vi "Bundle Script_Cluster Terminal Bundle.vi"(4 "Hide Full Names":bool=TRUE, 6 "Object Placement":enum32{"Choice 1", "Choice 2"}(radio), 8 "error in":errorcluster, 10 "Selected Items Tags":string[](array[string]), 11 "Affected Items":T1) -> (0 "error out":errorcluster, 2 "Objects":refnum<vi>[](array[refnum]))   [LabVIEW 2023]
uses:
  top/BundleMagic.ctl
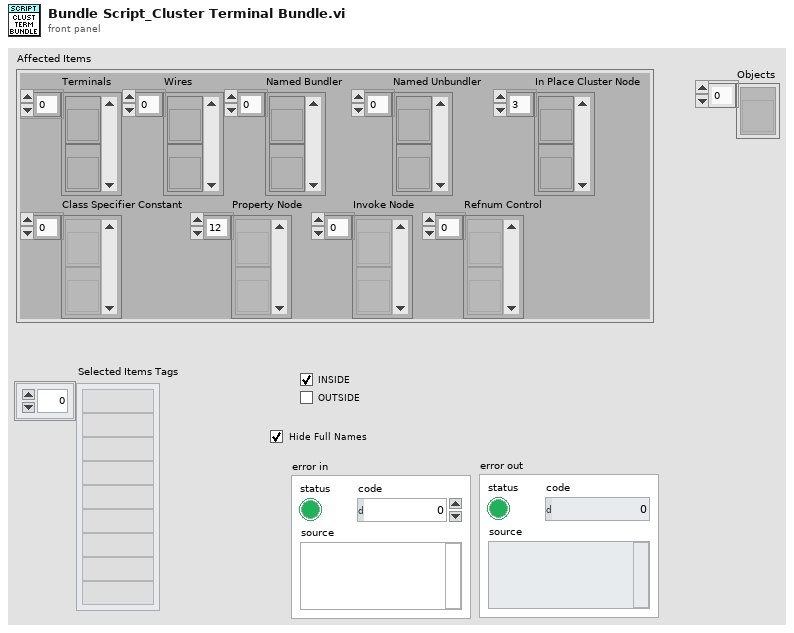
[diagram p1: front panel]
types:
  T1 = typedef "BundleMagic.ctl" = cluster{"Terminals":refnum<vi>[], "Wires":refnum<vi>[], "Named Bundler":refnum<vi>[], "Named Unbundler":refnum<vi>[], "In Place Cluster Node":refnum<vi>[], "Class Specifier Constant":refnum<vi>[], "Property Node":refnum<vi>[], "Invoke Node":refnum<vi>[], "Refnum Control":refnum<vi>[]}
  T2 = enum32{"Top Edges", "Vertical Centers", "Bottom Edges", "Left Edges", "Horizontal Centers", "Right Edges"}
  T3 = cluster{"Tunnel Ref":refnum<vi>, "On Tunnel?":bool, "Placement":enum32{"Choice 1", "Choice 2"}, "Tunnel Is Indexing?":bool, "Diagram":refnum<vi>, "Position":cluster{"Refnum":refnum<vi>, "Relative Direction":enum32{"Right", "Left", "Top", "Bottom", "Top Right", "Top Left", "Bottom Right", "Bottom Left"}, "Point32":cluster{"Horizontal":i32, "Vertical":i32}}, "Chosen Terminal":refnum<vi>, "Is Refnum?":bool, "Is Cluster?":bool, "Is Source?":bool, "Tunnel Direction":enum16{"In-Going", "Out-Going"}, "Tunnel Position":enum16{"Left", "Top", "Right", "Bottom"}, "Is Inner?":bool, "Terminal Is Indexing?":bool}
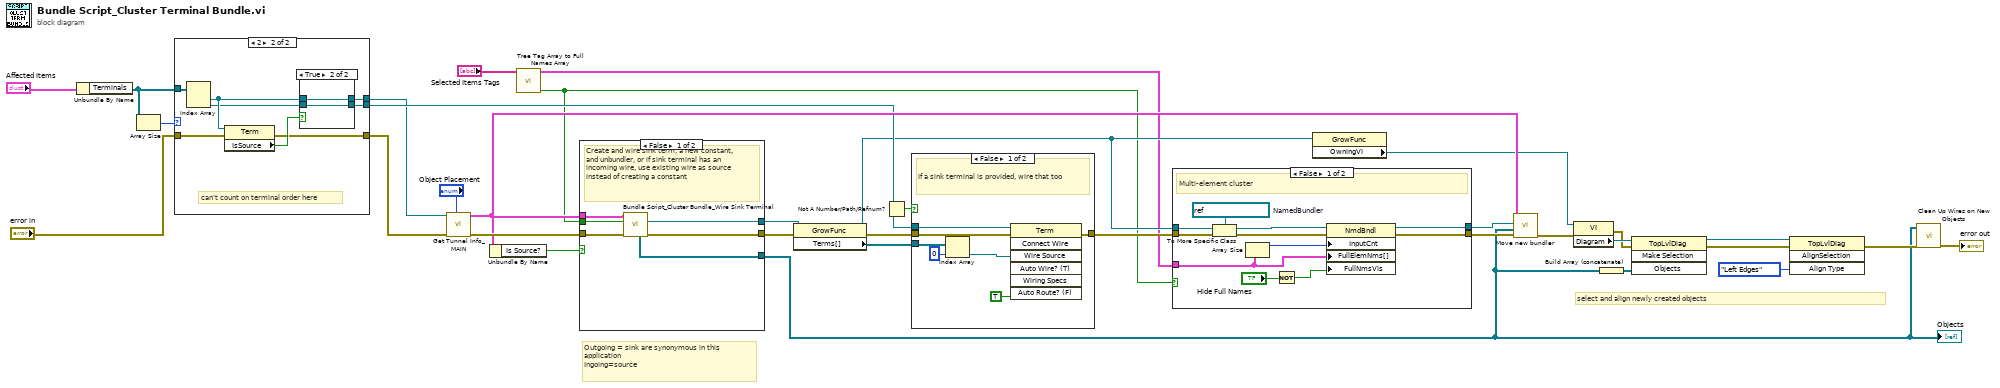
[diagram p0: block diagram]
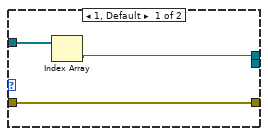
[diagram p2: hidden frame]
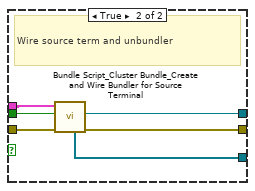
[diagram p4: hidden frame]
diagram:
  # "Outgoing = sink are synonymous in this application\nIngoing=source"
  # "select and align newly created objects"
  n1 = Unbundle By Name("Affected Items") -> ("Terminals"=w14:refnum<vi>[])
  n2 = Array Size(array=w14) -> (size(s)=w13:i32)
  n3 = case shown="2" w13 {
    tunnel: w14 -> [w37 w45]
    tunnel: [w36 w42] -> w4
    tunnel: [_ w40] -> w15
    tunnel: "error in" -> [w35 w39]
    tunnel: [w35 w38] -> w5
    frame 1, Default {
      n4 = Index Array(array=w37) -> (element=w36:refnum<vi>)  [unwired: 1 in]
    }
    frame 2 {
      # "can't count on terminal order here"
      n5 = Index Array(array=w45) -> (element #1=w43:refnum<vi>, element #2=w41:refnum<vi>)  [unwired: 2 in]
      n6 = property class="Term"(reference=w43, error in=w39) -> (error out=w38:errorcluster, "IsSource"=w44:bool)  [unwired: 1 out]
      n7 = case shown="True" w44 {
        tunnel: [w46 w49] -> w42
        tunnel: w43 -> [w47 w49]
        tunnel: [w47 w48] -> w40
        tunnel: w41 -> [w46 w48]
        frame False {
        }
        frame True {
        }
      }
    }
  }
  n8 = call "Get Tunnel Info_MAIN.vi"("Object Placement"="Object Placement", "error in"=w5, "Terminal in"=w4) -> ("error out"=w25:errorcluster, "Terminal Data Cluster"=w16:T3)  [unwired: 6 in, 1 out]
  n9 = Unbundle By Name(w16) -> ("Is Source?"=w24:bool)
  n10 = call "Tree Tag Array to Full Names Array.vi"("Selected Items Tags"="Selected Items Tags") -> ("Unnamed?"=w1:bool, "Tree Item Values (nested form)"=w2:cluster{"Array":string[]}[])  [unwired: 6 in, 3 out]
  n11 = case shown="False" w24 {
    tunnel: [w54 w60] -> w30
    tunnel: w25 -> [w55 w61]
    tunnel: [w53 w59] -> w31
    tunnel: [w52 w58] -> w10
    tunnel: w16 -> [w51 w57]
    tunnel: w1 -> [w50 w56]
    frame False {
      # "Create and wire sink term, a new constant, and unbundler, or if sink terminal has an incoming wire, use existing wire as source instead of creating a constant"
      n12 = call "Bundle Script_Cluster Bundle_Wire Sink Terminal.vi"("error in"=w55, "Unnamed?"=w50, "Tunnel Data Cluster"=w51) -> ("error out"=w54:errorcluster, "Bundler Refnum"=w53:refnum<vi>, "New objects created"=w52:refnum<vi>[])  [unwired: 6 in]
    }
    frame True {
      # "Wire source term and unbundler"
      n13 = call "Bundle Script_Cluster Bundle_Create and Wire Bundler for Source Terminal.vi"("error in"=w61, "Unnamed?"=w56, "Tunnel Data Cluster"=w57) -> ("error out"=w60:errorcluster, "Bundler Refnum"=w59:refnum<vi>, "New objects created"=w58:refnum<vi>[])  [unwired: 6 in]
    }
  }
  "Objects" <- w10
  n14 = property class="GrowFunc"(reference=w31, error in=w30) -> (reference out=w9:refnum<vi>, error out=w29:errorcluster, "Terms[]"=w32:refnum<vi>[])
  n15 = Not A Number/Path/Refnum?(number/path/refnum=w15) -> (NaN/Path/Refnum?=w33:bool)
  n16 = case shown="False" w33 {
    tunnel: w29 -> [w68 w69]
    tunnel: [w67 w69] -> w34
    tunnel: w32 -> [w65 _]
    tunnel: w15 -> [w63 _]
    frame False {
      # "If a sink terminal is provided, wire that too"
      n17 = Index Array(array=w65, index=0) -> (element=w62:refnum<vi>)
      n18 = invoke class="Term" method="Connect Wire"(reference=w63, error in=w68, "Wire Source"=w62, "Auto Route? (F)"=TRUE) -> (error out=w67:errorcluster)  [unwired: 3 in, 6 out]
    }
    frame True {
    }
  }
  n19 = case shown="False" w1 {
    tunnel: w34 -> [w75 w81]
    tunnel: [w79 w81] -> w19
    tunnel: [w78 w82] -> w17
    tunnel: w2 -> [w72 _]
    tunnel: w9 -> [w74 w82]
    frame False {
      w73 = refnum<vi> refnum  # NamedBundler
      # "Multi-element cluster"
      n20 = To More Specific Class(target class=w73, reference=w74, error in=w75) -> (specific class reference=w77:refnum<vi>, error out=w76:errorcluster)
      n21 = Array Size(array=w72) -> (size(s)=w80:i32)
      n22 = Not(x="Hide Full Names") -> (.not. x?=w70:bool)
      n23 = property class="NmdBndl"(reference=w77, error in=w76, "InputCnt"=w80, "FullElemNms[]"=w72, "FullNmsVis"=w70) -> (reference out=w78:refnum<vi>, error out=w79:errorcluster)
    }
    frame True {
      # "when dropped the single element cluster will assume the correct element count, so nothing to do here"
      # "Single-element cluster"
    }
  }
  n24 = property class="GrowFunc"(reference=w9) -> ("OwningVI"=w8:refnum<vi>)  [unwired: 1 in, 2 out]
  n25 = call "Move new bundler.vi"("error in"=w19, "New objects created"=w10, "Named Un/Bundler Ref"=w17, "Tunnel Data Cluster"=w16) -> ("error out"=w18:errorcluster)  [unwired: 7 in]
  n26 = property class="VI"(reference=w8, error in=w18) -> (error out=w27:errorcluster, "Diagram"=w28:refnum<vi>)  [unwired: 1 out]
  n27 = Build Array (concatenate)(w10) -> (w26:refnum<vi>[])
  n28 = invoke class="TopLvlDiag" method="Make Selection"(reference=w28, error in=w27, "Objects"=w26) -> (reference out=w21:refnum<vi>, error out=w20:errorcluster)  [unwired: 1 in, 2 out]
  n29 = invoke class="TopLvlDiag" method="AlignSelection"(reference=w21, error in=w20, "Align Type"=T2."Left Edges") -> (error out=w12:errorcluster)  [unwired: 1 in, 3 out]
  n30 = call "Clean Up Wires on New Objects.vi"("error in (no error)"=w12, "New objects created"=w10) -> ("error out"=→"error out":errorcluster)  [unwired: 9 in]
